vi "myXi_SetParameter.vi"(6 "input value DBL":sgl, 7 "input PRM":T2, 8 "error in":errorcluster, 9 "input value I32":i64, 11 "xiCam IN":refnum<k24>) -> (0 "error out":errorcluster, 3 "xiCam Out":refnum<k24>)   [LabVIEW 2018]
uses:
  VisionLibrariesXimea/xiLib/xiLIB_64bit/xiLIB/xiCamLib/xiCam/PRM/PRM/PRM_v2.ctl
  C:/XIMEA/API/x64/xiApi.NETX64.dll
  VisionLibrariesXimea/xiLib/xiLIB_64bit/xiLIB/xiCamLib/xiLIB/Typedefs/xiLIB - PRM_Type.ctl
panel:
  out "Type":T1
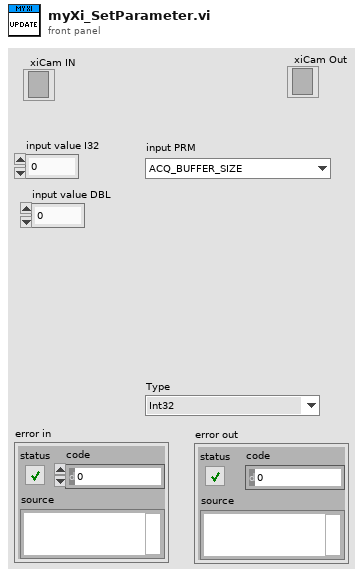
[diagram p1: front panel]
types:
  T1 = typedef "xiLIB - PRM_Type.ctl" = enum16{"Int32", "Float", "String", "DOWNSAMPLING_TYPE", "IMAGE_DATA_FORMAT", "BUFFER_POLICY", "TRG_SOURCE", "GPI", "GPO", "ACQ_TIMING_MODE", "BINNING_PATTERN", "BINNING_SELECTOR", "CMS_MODE", "COUNTER_SELECTOR", "DEBUG_LEVEL", "DECIMATION_PATTERN", "DECIMATION_SELECTOR", "GAIN_SELECTOR_TYPE", "LED_MODE", "LENS_FEATURE_SELECTOR", "LENS_MODE", "OUTPUT_DATA_PACKING_TYPE", "SENSOR_FEATURE_SELECTOR", "SHUTTER_TYPE", "TRG_SELECTOR", "TS_RST_MODE", "TS_RST_SOURCE"}
  T2 = typedef "PRM_v2.ctl" = enum16{"ACQ_BUFFER_SIZE", "ACQ_FRAME_BURST_COUNT", "ACQ_TIMING_MODE", "ACQ_TRANSPORT_BUFFER_SIZE", "AE_MAX_LIMIT", "AEAG", "AEAG_LEVEL", "API_VERSION", "AG_MAX_LIMIT", "APPLY_CMS", "AUTO_BANDWIDTH_CALCULATION", "AUTO_WB", "AVAILABLE_BANDWIDTH", "AVAILABLE_BANDWIDTH_MAX", "AVAILABLE_BANDWIDTH_MIN", "BPC", "BUFFER_POLICY", "BUFFERS_QUEUE_SIZE", "CC_MATRIX_00", "CC_MATRIX_01", "CC_MATRIX_02", "CC_MATRIX_03", "CC_MATRIX_10", "CC_MATRIX_11", "CC_MATRIX_12", "CC_MATRIX_13", "CC_MATRIX_20", "CC_MATRIX_21", "CC_MATRIX_22", "CC_MATRIX_23", "CC_MATRIX_30", "CC_MATRIX_31", "CC_MATRIX_32", "CC_MATRIX_33", "CHIP_TEMP", "CMS", "COLOR_FILTER_ARRAY", "COOLING", "DEBOUNCE_EN", "DEBOUNCE_POL", "DEBOUNCE_T0", "DEBOUNCE_T1", "DEBUG_LEVEL", "DEFAULT_CC_MATRIX", "DEVICE_INSTANCE_PATH", "DEVICE_MODEL_ID", "DEVICE_NAME", "DEVICE_SN", "DEVICE_TYPE", "DEVICE_USER_ID", "DOWNSAMPLING", "DOWNSAMPLING_MAX", "DOWNSAMPLING_MIN", "DOWNSAMPLING_TYPE", "DRV_VERSION", "EXP_PRIORITY", "EXPOSURE", "EXPOSURE_DIRECT_UPDATE", "EXPOSURE_MAX", "EXPOSURE_MIN", "FFS_FILE_NAME", "FPGA1_VERSION", "FRAMERATE", "FRAMERATE_MAX", "FRAMERATE_MIN", "FREE_FFS_SIZE", "GAIN", "GAIN_DIRECT_UPDATE", "GAIN_MAX", "GAIN_MIN", "GAMMAC", "GAMMAY", "GPI_LEVEL", "GPI_MODE", "GPI_SELECTOR", "GPI_SELECTOR_MAX", "GPI_SELECTOR_MIN", "GPO_MODE", "GPO_SELECTOR", "GPO_SELECTOR_MAX", "GPO_SELECTOR_MIN", "HDR", "HDR_T1", "HDR_T2", "HEIGHT", "HEIGHT_MAX", "HEIGHT_MIN", "HOUSE_TEMP", "IMAGE_DATA_FORMAT", "IMAGE_IS_COLOR", "INPUT_CMS_PROFILE", "IS_COOLED", "IS_DEVICE_EXIST", "KNEEPOINT1", "KNEEPOINT2", "LED_MODE", "LED_SELECTOR", "LED_SELECTOR_MAX", "LED_SELECTOR_MIN", "LIMIT_BANDWIDTH", "LIMIT_BANDWIDTH_MAX", "LIMIT_BANDWIDTH_MIN", "LUT_EN", "LUT_INDEX", "LUT_INDEX_MAX", "LUT_INDEX_MIN", "LUT_VALUE", "LUT_VALUE_MAX", "LUT_VALUE_MIN", "MANUAL_WB", "MCU1_VERSION", "MCU2_VERSION", "OFFSET_X", "OFFSET_X_MAX", "OFFSET_X_MIN", "OFFSET_Y", "OFFSET_Y_MAX", "OFFSET_Y_MIN", "OUTPUT_CMS_PROFILE", "OUTPUT_DATA_BIT_DEPTH", "OUTPUT_DATA_PACKING", "READ_FILE_FFS", "RECENT_FRAME", "SENSOR_DATA_BIT_DEPTH", "SENSOR_MODE", "SENSOR_TAPS", "SHARPNESS", "SHUTTER_TYPE", "TARGET_TEMP", "TRG_DELAY", "TRG_SELECTOR", "TRG_SOFTWARE", "TRG_SOURCE", "USED_FFS_SIZE", "WB_KB", "WB_KG", "WB_KR", "WIDTH", "WIDTH_MAX", "WIDTH_MIN", "WRITE_FILE_FFS", "ACQ_BUFFER_SIZE_UNIT", "ACQ_TRANSPORT_BUFFER_COMMIT", "AEAG_ROI_HEIGHT", "AEAG_ROI_OFFSET_X", "AEAG_ROU_OFFSET_Y", "AEAG_ROI_WIDTH", "API_CONTEXT_LIST", "BINNING_HORIZONTAL", "BINNING_SELECTOR", "BINNING_VERTICAL", "COLUMN_FPN_CORRECTION", "COUNTER_SELECTOR", "COUNTER_VALUE", "DECIMATION_HORIZONTAL", "DECIMATION_SELECTOR", "DECIMATION_VERTICAL", "DEVICE_ID", "DEVICE_LOCATION_PATH", "DEVICE_MANIFEST", "DEVICE_RESET", "DEVICE_SENS_SN", "EXPOSURE_BURST_COUNT", "FFS_ACCESS_KEY", "GAIN_SELECTOR", "HW_REVISION", "IMAGE_BLACK_LEVEL", "IMAGE_DATA_BIT_DEPTH", "IMAGE_DATA_FORMAT_RGB32_ALPHA", "IMAGE_PAYLOAD_SIZE", "LENS_APERTURE_VALUE", "LENS_FEATURE", "LENS_FEATURE_SELECTOR", "LENS_FOCAL_LENGTH", "LENS_FOCUS_DISTANCE", "LENS_FOCUS_MOVE", "LENS_FOCUS_MOVEMENT_VALUE", "LENS_MODE", "OUTPUT_DATA_PACKING_TYPE", "SENSOR_CLOCK_FREQ_HZ", "SENSOR_CLOCK_FREQ_INDEX", "SENSOR_FEATURE_SELECTOR", "SENSOR_FEATURE_VALUE", "SENSOR_OUTPUT_CHANNEL_COUNT", "TRANSPORT_PIXEL_FORMAT", "TS_RST_MODE", "TS_RST_SOURCE"}
  T3 = typedef "xiLIB - PRM_Attribute.ctl" = cluster{"Type":T1, "Method":T4, "Desc.":string, "PRM":T2}
  T4 = typedef "xiLIB - PRM_Function.ctl" = enum16{"Get / Set", "Get", "Set"}
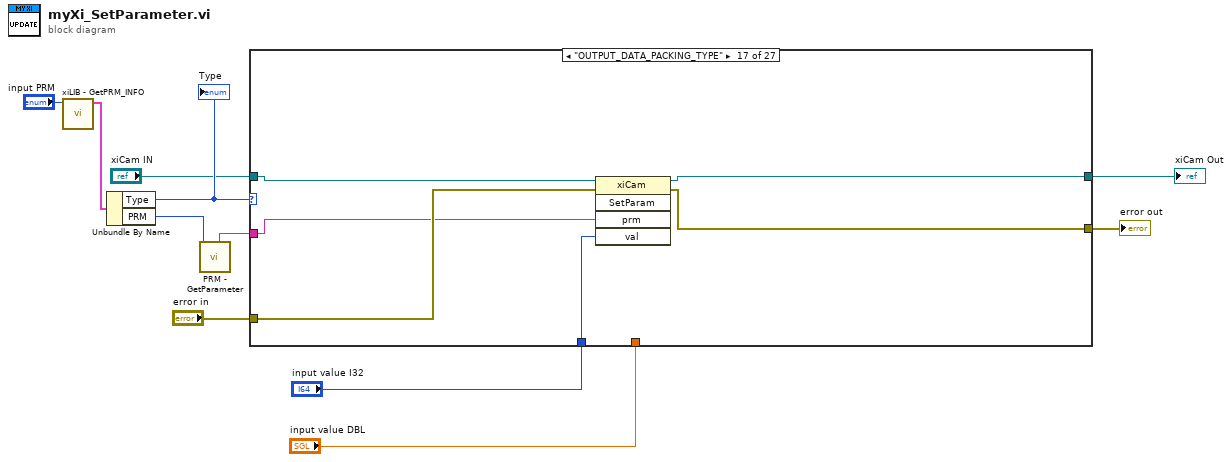
[diagram p0: block diagram]
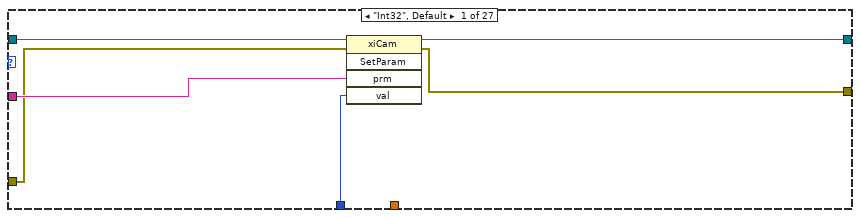
[diagram p2: hidden frame]
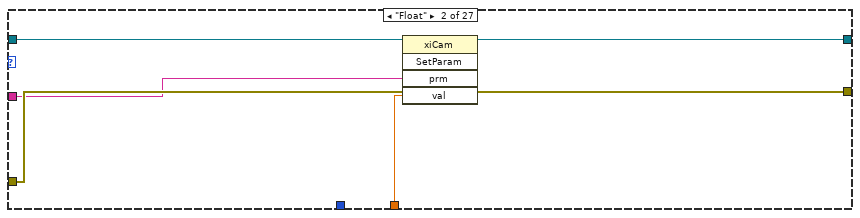
[diagram p3: hidden frame]
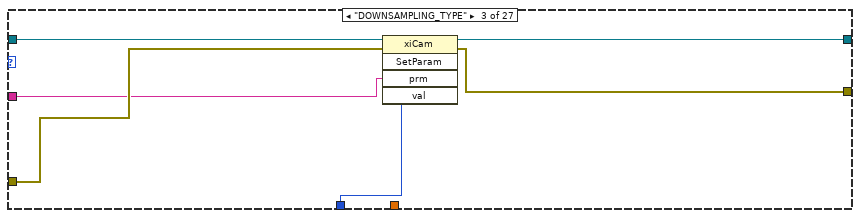
[diagram p4: hidden frame]
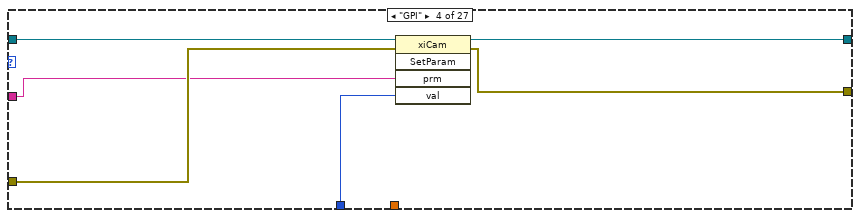
[diagram p5: hidden frame]
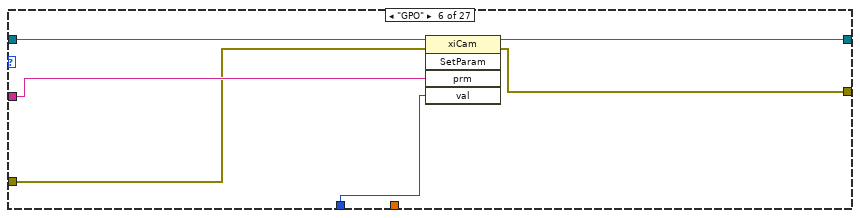
[diagram p7: hidden frame]
diagram:
  n1 = call "xiLIB - GetPRM_INFO.vi"("PRM"="input PRM") -> ("PRM_Attributes"=w10:T3)  [unwired: 10 in]
  n2 = Unbundle By Name(w10) -> ("Type"=w9:T1, "PRM"=w4:T2)
  "Type" <- w9
  n3 = call "PRM - GetParameter.vi"("PRM"=w4) -> ("ParameterString"=w3:string)  [unwired: 8 in, 2 out]
  n4 = case shown="\"OUTPUT_DATA_PACKING_TYPE\"" w9 {
    tunnel: "xiCam IN" -> [w16 w21 w28 w33 w36 w42 w44 w46 w48 w50 w52 w54 w56 w58 w60 w62 w68 w70 w72 w74 w76 w78 w84 w86 w92 w94 w96]
    tunnel: [w15 w20 w27 w32 w36 w41 w44 w46 w48 w50 w52 w54 w56 w58 w60 w62 w67 w70 w72 w74 w76 w78 w83 w86 w90 w94 w96] -> w7
    tunnel: [w14 w22 w26 w31 w35 w40 w43 w45 w47 w49 w51 w53 w55 w57 w59 w61 w63 w69 w71 w73 w75 w77 w81 w85 w89 w93 w95] -> w6
    tunnel: "error in" -> [w13 w22 w25 w34 w35 w37 w43 w45 w47 w49 w51 w53 w55 w57 w59 w61 w66 w69 w71 w73 w75 w77 w82 w85 w91 w93 w95]
    tunnel: w3 -> [w17 w19 w24 w30 _ w38 _ _ _ _ _ _ _ _ _ _ w64 _ _ _ _ _ w80 _ w88 _ _]
    tunnel: "input value I32" -> [w12 _ w23 w29 _ w39 _ _ _ _ _ _ _ _ _ _ w65 _ _ _ _ _ w79 _ w87 _ _]
    tunnel: "input value DBL" -> [_ w18 _ _ _ _ _ _ _ _ _ _ _ _ _ _ _ _ _ _ _ _ _ _ _ _ _]
    frame "Int32", Default {
      n5 = invoke class="xiCam" method="SetParam"(reference=w16, error in=w13, "prm"=w17, "val"=w12) -> (reference out=w15:refnum<k24>, error out=w14:errorcluster)  [unwired: 1 in, 3 out]
    }
    frame "Float" {
      n6 = invoke class="xiCam" method="SetParam"(reference=w21, "prm"=w19, "val"=w18) -> (reference out=w20:refnum<k24>)  [unwired: 2 in, 4 out]
    }
    frame "DOWNSAMPLING_TYPE" {
      n7 = invoke class="xiCam" method="SetParam"(reference=w28, error in=w25, "prm"=w24, "val"=w23) -> (reference out=w27:refnum<k24>, error out=w26:errorcluster)  [unwired: 1 in, 3 out]
    }
    frame "GPI" {
      n8 = invoke class="xiCam" method="SetParam"(reference=w33, error in=w34, "prm"=w30, "val"=w29) -> (reference out=w32:refnum<k24>, error out=w31:errorcluster)  [unwired: 1 in, 3 out]
    }
    frame "CMS_MODE" {
    }
    frame "GPO" {
      n9 = invoke class="xiCam" method="SetParam"(reference=w42, error in=w37, "prm"=w38, "val"=w39) -> (reference out=w41:refnum<k24>, error out=w40:errorcluster)  [unwired: 1 in, 3 out]
    }
    frame "String" {
    }
    frame "ACQ_TIMING_MODE" {
    }
    frame "COUNTER_SELECTOR" {
    }
    frame "DEBUG_LEVEL" {
    }
    frame "DECIMATION_PATTERN" {
    }
    frame "DECIMATION_SELECTOR" {
    }
    frame "GAIN_SELECTOR_TYPE" {
    }
    frame "LED_MODE" {
    }
    frame "LENS_FEATURE_SELECTOR" {
    }
    frame "LENS_MODE" {
    }
    frame "OUTPUT_DATA_PACKING_TYPE" {
      n10 = invoke class="xiCam" method="SetParam"(reference=w68, error in=w66, "prm"=w64, "val"=w65) -> (reference out=w67:refnum<k24>, error out=w63:errorcluster)  [unwired: 1 in, 3 out]
    }
    frame "SENSOR_FEATURE_SELECTOR" {
    }
    frame "SHUTTER_TYPE" {
    }
    frame "TRG_SELECTOR" {
    }
    frame "TS_RST_MODE" {
    }
    frame "TS_RST_SOURCE" {
    }
    frame "IMAGE_DATA_FORMAT" {
      n11 = invoke class="xiCam" method="SetParam"(reference=w84, error in=w82, "prm"=w80, "val"=w79) -> (reference out=w83:refnum<k24>, error out=w81:errorcluster)  [unwired: 1 in, 3 out]
    }
    frame "BUFFER_POLICY" {
    }
    frame "TRG_SOURCE" {
      n12 = invoke class="xiCam" method="SetParam"(reference=w92, error in=w91, "prm"=w88, "val"=w87) -> (reference out=w90:refnum<k24>, error out=w89:errorcluster)  [unwired: 1 in, 3 out]
    }
    frame "BINNING_PATTERN" {
    }
    frame "BINNING_SELECTOR" {
    }
  }
  "xiCam Out" <- w7
  "error out" <- w6
